vi "calculate best match.vi"(9 "Array":bool[][](array[boolean]), 10 "Allowed columns":bool[](array[boolean]), 11 "comparison":bool[](array[boolean])) -> (0 "Acceptable solution":bool, 1 "rank":i32, 2 "other index":i32, 3 "Result":bool[](array[boolean]))   [LabVIEW 2009]
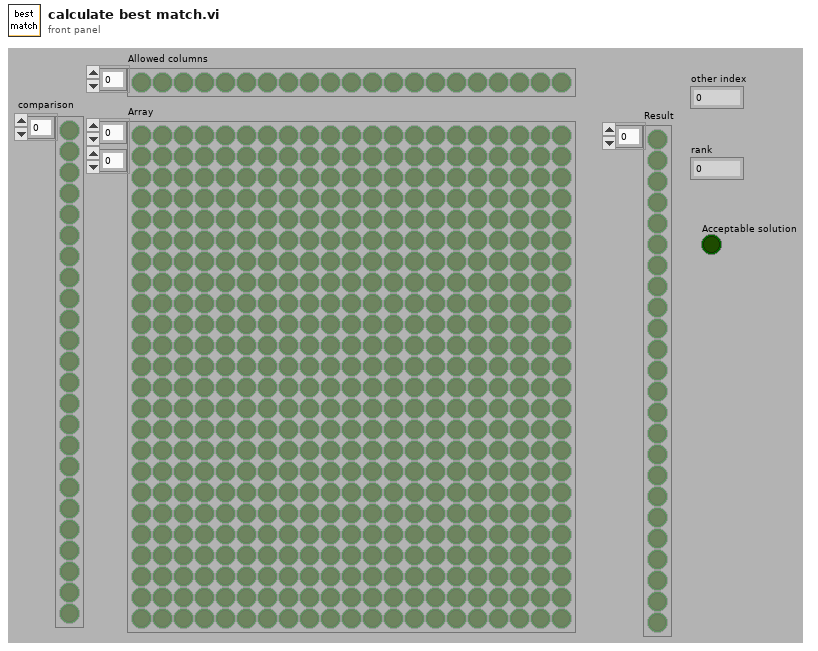
[diagram p1: front panel]
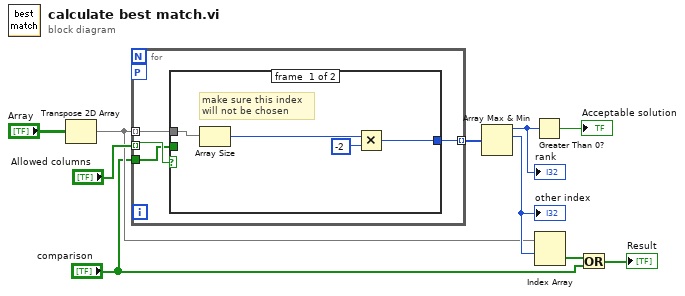
[diagram p0: block diagram]
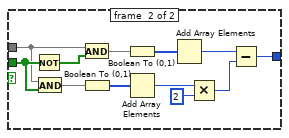
[diagram p2: hidden frame]
diagram:
  n1 = Transpose 2D Array(2D array="Array") -> (transposed array=w4:bool[][])
  n2 = for {
    tunnel: w4 -> [w13] mode=indexing
    tunnel: "Allowed columns" -> [w14] mode=indexing
    tunnel: "comparison" -> [w12]
    tunnel: [w11] -> w8 mode=indexing
    workers-P: _ -> [_]
    n3 = case shown="True" w14 {
      tunnel: w13 -> [w18 w29]
      tunnel: w12 -> [_ w30]
      tunnel: [w15 w20] -> w11
      frame #0 {
        # "make sure this index\nwill not be chosen"
        n4 = Array Size(array=w18) -> (size(s)=w17:i32)
        n5 = Multiply(x=w17, y=-2) -> (x*y=w15:i32)
      }
      frame #1 {
        n6 = Not(x=w30) -> (.not. x?=w19:bool[])
        n7 = And(x=w29, y=w30) -> (x .and. y?=w28:bool[])
        n8 = And(x=w29, y=w19) -> (x .and. y?=w27:bool[])
        n9 = Boolean To (0,1)(Boolean=w28) -> (0, 1=w25:i16[])
        n10 = Boolean To (0,1)(Boolean=w27) -> (0, 1=w26:i16[])
        n11 = Add Array Elements(numeric array=w25) -> (sum=w24:i16)
        n12 = Add Array Elements(numeric array=w26) -> (sum=w21:i16)
        n13 = Multiply(x=w24, y=i16 2) -> (x*y=w22:i16)
        n14 = Subtract(x=w21, y=w22) -> (x-y=w20:i16)
      }
    }
  }
  n15 = Array Max & Min(array=w8) -> (max value=w7:i32, max index (indices)=w5:i32)  [unwired: 2 out]
  "other index" <- w5
  "rank" <- w7
  n16 = Greater Than 0?(x=w7) -> (x > 0?=→"Acceptable solution":bool)
  n17 = Index Array(array=w4, index (row)=w5) -> (element=w3:bool[])  [unwired: 1 in]
  n18 = Or(x=w3, y="comparison") -> (x .or. y?=→"Result":bool[])
